vi "DiffDriveSim_CreateCustomDrive.vi"(4 "Skid Factor":dbl=1.75, 6 "Actual TrackWidth Inch":dbl=21.0 format="%#_13g", 8 "Measurement StdDev":T3, 9 "Custom Drive Info":T5 {"Gear Ratio" format="%#_13g"; "Wheel Diameter Inch" format="%#_13g"}, 10 "j_KgM2":dbl, 11 "Mass_LB":dbl) -> (2 "Meters":dbl, 3 "DiffDriveTrainSim":T1 {"m_Motor"."Jr_KgM2" format="%13.5p"; "m_Motor"."L_H" format="%13.5p"; "m_Motor"."Kt_NMPerAmp" format="%13.5p"; "m_Motor"."KvINV_RadPerSecPerVolt" format="%13.5p"; "m_Motor"."R_Ohms" format="%13.5p"; "m_Motor"."FreeSpeed_RadPerSec" format="%13.5p"; "m_Motor"."FreeCurrent_Amps" format="%13.5p"; "m_Motor"."StallCurrent_Amps" format="%13.5p"; "m_Motor"."StallTorque_NM" format="%13.5p"; "m_Motor"."nominalVoltage_Volts" format="%13.5p"})   [LabVIEW 2019]
uses:
  DiffDriveSim_CustomDriveIntoType.ctl
  <vilib>/Rock Robotics/WPI/ThirdParty/JAS_Junk/TrajLib/Enum/DCMOTOR_TYPES_ENUM.ctl
  <vilib>/Analysis/Matrix/Datatypes/RealMatrix.ctl
  <vilib>/Rock Robotics/WPI/ThirdParty/JAS_Junk/TrajLib/TypeDef/DIFF_DRIVE_TRAIN_SIM.ctl
  <vilib>/Rock Robotics/WPI/ThirdParty/JAS_Junk/TrajLib/TypeDef/LINEAR_SYSTEM.ctl
  <vilib>/Rock Robotics/WPI/ThirdParty/JAS_Junk/TrajLib/TypeDef/DCMOTOR.CTL
  <vilib>/Rock Robotics/WPI/ThirdParty/JAS_Junk/TrajLib/DCMotor_GetCIM.vi
  <vilib>/Rock Robotics/WPI/ThirdParty/JAS_Junk/TrajLib/DCMotor_GetAndymark9015.vi
  <vilib>/Rock Robotics/WPI/ThirdParty/JAS_Junk/TrajLib/DCMotor_GetAndymarkRs775_125.vi
  <vilib>/Rock Robotics/WPI/ThirdParty/JAS_Junk/TrajLib/DCMotor_GetBag.vi
  <vilib>/Rock Robotics/WPI/ThirdParty/JAS_Junk/TrajLib/DCMotor_GetBanebotsRs550.vi
  <vilib>/Rock Robotics/WPI/ThirdParty/JAS_Junk/TrajLib/DCMotor_GetBanebotsRs775.vi
  <vilib>/Rock Robotics/WPI/ThirdParty/JAS_Junk/TrajLib/DCMotor_GetFalcon500.vi
  <vilib>/Rock Robotics/WPI/ThirdParty/JAS_Junk/TrajLib/DCMotor_GetMiniCIM.vi
  <vilib>/Rock Robotics/WPI/ThirdParty/JAS_Junk/TrajLib/DCMotor_GetNEO.vi
  <vilib>/Rock Robotics/WPI/ThirdParty/JAS_Junk/TrajLib/DCMotor_GetNEO550.vi
  <vilib>/Rock Robotics/WPI/ThirdParty/JAS_Junk/TrajLib/DCMotor_GetRomiBuiltIn.vi
  <vilib>/Rock Robotics/WPI/ThirdParty/JAS_Junk/TrajLib/DCMotor_GetVex775Pro.vi
  <vilib>/Rock Robotics/WPI/ThirdParty/JAS_Junk/TrajLib/LinearSystem_New.vi
  <vilib>/Rock Robotics/WPI/ThirdParty/JAS_Junk/TrajLib/MatBuilder_Create.vi
  <vilib>/Rock Robotics/WPI/ThirdParty/JAS_Junk/TrajLib/MatBuilder_Fill.vi
  <vilib>/Rock Robotics/WPI/ThirdParty/JAS_Junk/TrajLib/MatrixHelper_Zero.vi
  <vilib>/Rock Robotics/WPI/ThirdParty/JAS_Junk/TrajLib/DCMotor_New.vi
  <vilib>/Rock Robotics/WPI/ThirdParty/JAS_Junk/TrajLib/VI/Units_RotationsPerMinuteToRadiansPerSecond.vi
  <vilib>/Rock Robotics/WPI/ThirdParty/JAS_Junk/TrajLib/MatrixHelper_CoerceSize.vi
  <vilib>/Rock Robotics/WPI/ThirdParty/JAS_Junk/TrajLib/Trajectory_Library.lvlib
  <vilib>/Analysis/Matrix/NI_Matrix.lvlib
panel:
  # "<States, 1>"
  # "<Outputs, 1>"
  # "<Inputs, 1>"
  # "<Outputs, 1>"
  # "<States,States>"
  # "<States,Inputs>"
  # "<Outputs,States>"
  # "<Outputs,Inputs>"
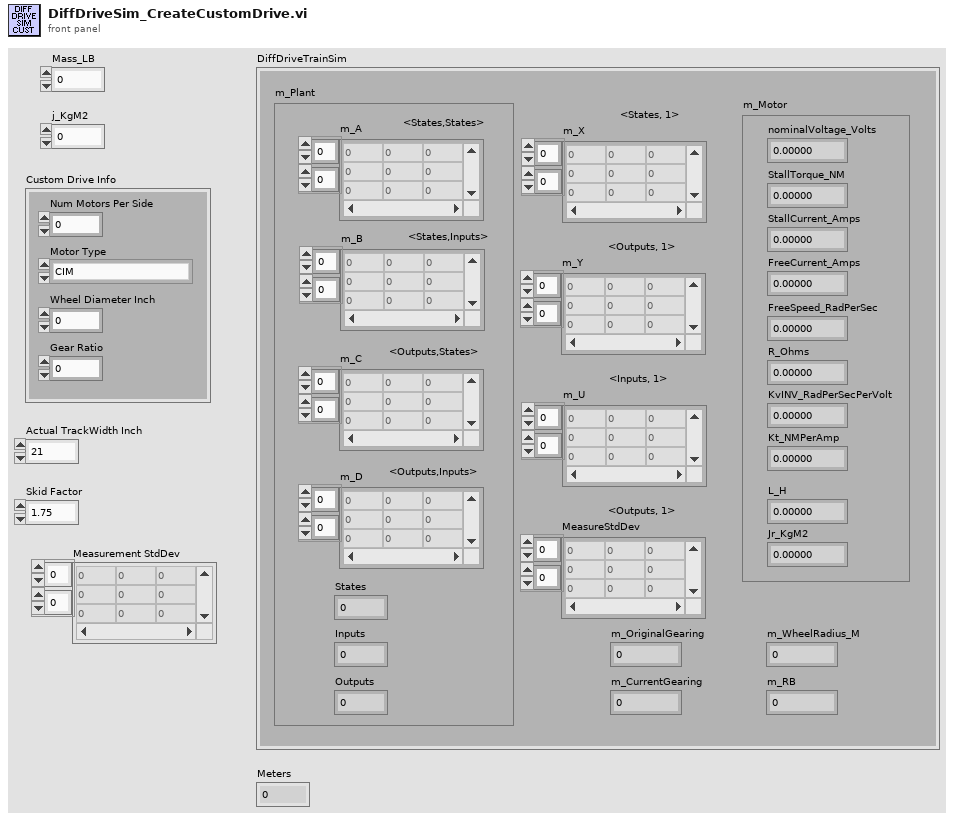
[diagram p1: front panel]
types:
  T1 = typedef "Trajectory_Library.lvlib/DIFF_DRIVE_TRAIN_SIM.ctl" = cluster{"m_Plant":T2, "m_X":T3, "m_Y":T3, "m_U":T3, "MeasureStdDev":T3, "m_Motor":T4, "m_OriginalGearing":dbl, "m_CurrentGearing":dbl, "m_WheelRadius_M":dbl, "m_RB":dbl}
  T2 = typedef "Trajectory_Library.lvlib/LINEAR_SYSTEM.ctl" = cluster{"m_A":T3, "m_B":T3, "m_C":T3, "m_D":T3, "States":i32, "Inputs":i32, "Outputs":i32}
  T3 = typedef "NI_Matrix.lvlib/RealMatrix.ctl" = dbl[][]
  T4 = typedef "Trajectory_Library.lvlib/DCMOTOR.CTL" = cluster{"nominalVoltage_Volts":dbl, "StallTorque_NM":dbl, "StallCurrent_Amps":dbl, "FreeCurrent_Amps":dbl, "FreeSpeed_RadPerSec":dbl, "R_Ohms":dbl, "KvINV_RadPerSecPerVolt":dbl, "Kt_NMPerAmp":dbl, "L_H":dbl, "Jr_KgM2":dbl}
  T5 = typedef "DiffDriveSim_CustomDriveIntoType.ctl" = cluster{"Motor Type":T6, "Num Motors Per Side":i32, "Wheel Diameter Inch":dbl, "Gear Ratio":dbl}
  T6 = typedef "Trajectory_Library.lvlib/DCMOTOR_TYPES_ENUM.ctl" = enum16{"CIM", "AndyMark 9015", "Andy Mark RS 775 125", "Bag", "BaneBots RS 550", "BaneBots RS 775", "Falcon 500", "Mini CIM", "NEO", "NEO 550", "Romi BuiltIn", "Vex 775 Pro"}
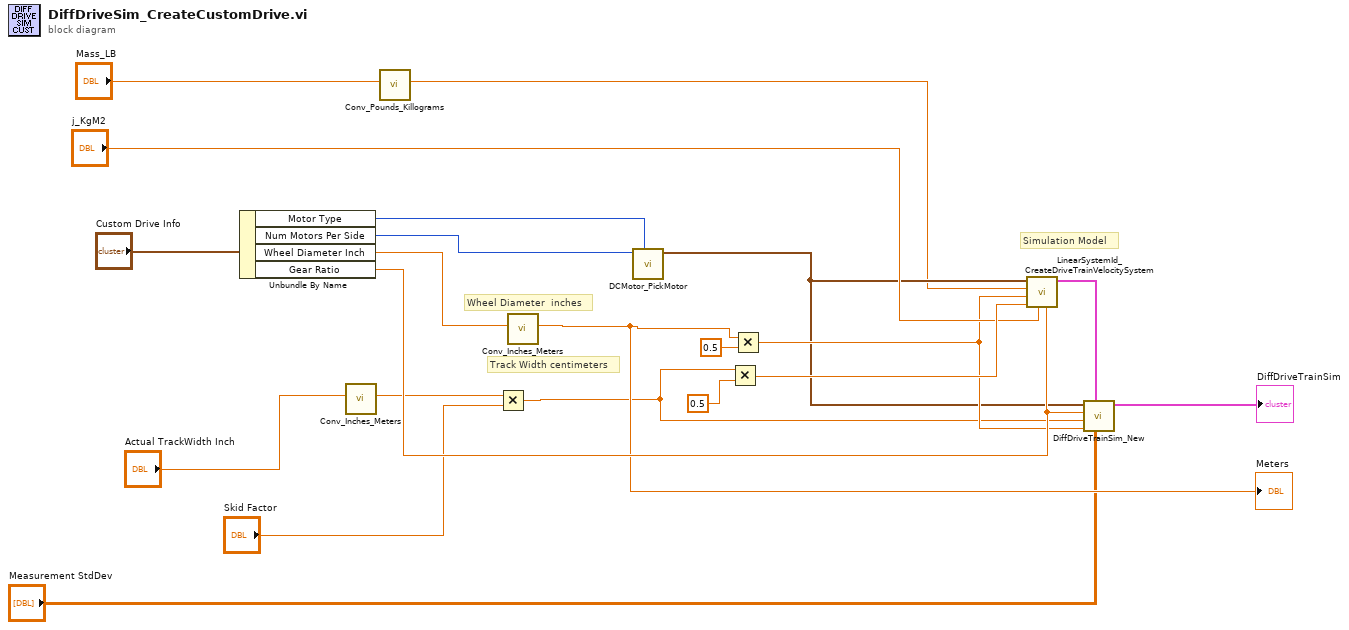
[diagram p0: block diagram]
diagram:
  # "Track Width centimeters"
  # "Wheel Diameter  inches"
  # "Simulation Model"
  n1 = Unbundle By Name("Custom Drive Info") -> ("Motor Type"=w18:T6, "Num Motors Per Side"=w19:i32, "Wheel Diameter Inch"=w20:dbl, "Gear Ratio"=w21:dbl)
  n2 = call <vilib>:"Conv_Inches_Meters.vi"("INCH"="Actual TrackWidth Inch") -> ("Meters"=w2:dbl)  [unwired: 10 in]
  n3 = call <vilib>:"Conv_Pounds_Killograms.vi"("Pounds"="Mass_LB") -> ("Killograms"=w5:dbl)  [unwired: 10 in]
  n4 = Multiply(x=w2, y="Skid Factor") -> (x*y=w1:dbl)
  n5 = call <vilib>:"Conv_Inches_Meters.vi"("INCH"=w20) -> ("Meters"=w16:dbl)  [unwired: 10 in]
  "Meters" <- w16
  n6 = call <vilib>:"DCMotor_PickMotor.vi"("DCMOTOR_TYPES"=w18, "Num Motors"=w19) -> ("DCMOTOR"=w9:T4)  [unwired: 9 in]
  n7 = Multiply(x=w1, y=0.5) -> (x*y=w13:dbl)
  n8 = Multiply(x=w16, y=0.5) -> (x*y=w11:dbl)
  n9 = call <vilib>:"LinearSystemId_CreateDriveTrainVelocitySystem.vi"("G"=w21, "JKgMetersSquared"="j_KgM2", "rbMeters"=w13, "rMeters"=w11, "MassKg"=w5, "Motor"=w9) -> ("Linearsystem"=w14:T2)  [unwired: 4 in, 1 out]
  n10 = call <vilib>:"DiffDriveTrainSim_New.vi"("MeasurementStdDev"="Measurement StdDev", "DriveTrainPlant"=w14, "WheelRadius_M"=w11, "TrackWidth_M"=w1, "Gearing"=w21, "DriveMotor"=w9) -> ("DiffDriveTrainSim"=→"DiffDriveTrainSim":T1)  [unwired: 5 in]
